vi "Configure RF Output.vi"(4 "Enable Reverse Power Protection (T:Enable)":bool=TRUE, 6 "Enable Blanking (T:Enable)":bool=TRUE, 7 "Enable Modulation (T:Enable)":bool=TRUE, 8 "error in (no error)":errorcluster, 9 "Auto Blanking (T:Enable)":bool=TRUE, 10 "Enable RF Output (F:Disable)":bool, 11 "VISA resource name":refnum<visa-resource-name>) -> (0 "error out":errorcluster, 3 "VISA resource name out":refnum<visa-resource-name>)   [LabVIEW 2012, in "Agilent PSG MXG Series.lvlib"]
doc: "Configures RF output, modulation state, blanking, and RPP circuit of the signal generator."
uses:
  <instrlib>/Agilent PSG MXG Series/Agilent PSG MXG Series.lvlib
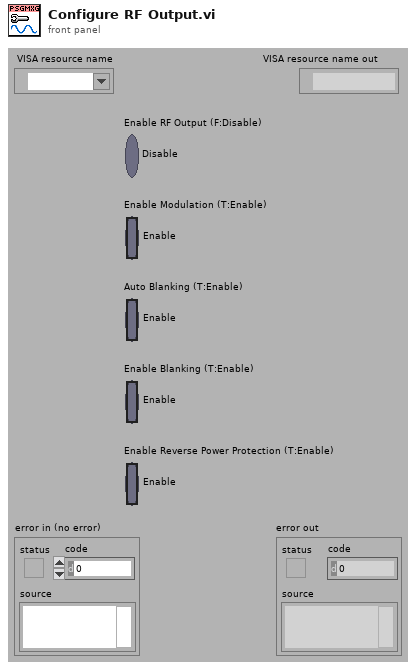
[diagram p1: front panel]
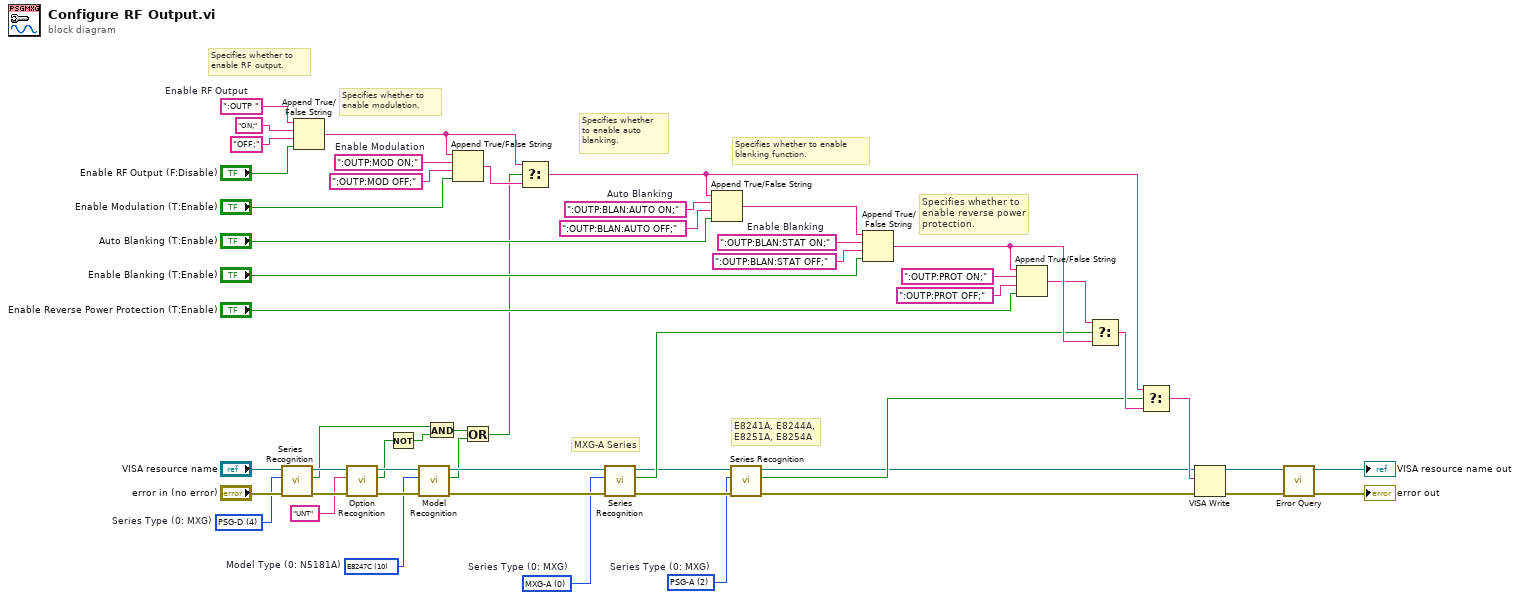
[diagram p0: block diagram]
diagram:
  w1 = u16 4 items=["MXG-A", "PSG", "PSG-A", "PSG-C", "PSG-D", "MXG-B", "EXG"]  # Series Type (0: MXG)
  w2 = u16 10 items=["N5181A"=0, "N5182A"=1, "N5183A"=2, "N5161A"=3, "N5162A"=4, "E8241A"=5, "E8244A"=6, "E8251A"=7, "E8254A"=8, "E8247C"=10, "E8257C"=11, "E8267C"=12, "E8257D"=15, "E8267D"=16, "N5171B"=17, "N5172B"=18, "N5181B"=19, "N5182B"=20]  # Model Type (0: N5181A)
  w3 = u16 2 items=["MXG-A", "PSG", "PSG-A", "PSG-C", "PSG-D", "MXG-B", "EXG"]  # Series Type (0: MXG)
  w4 = u16 0 items=["MXG-A", "PSG", "PSG-A", "PSG-C", "PSG-D", "MXG-B", "EXG"]  # Series Type (0: MXG)
  w31 = ":OUTP:BLAN:STAT ON;"  # Enable Blanking
  w46 = ":OUTP:BLAN:AUTO ON;"  # Auto Blanking
  w49 = ":OUTP:MOD ON;"  # Enable Modulation
  w53 = ":OUTP "  # Enable RF Output
  # "MXG-A Series"
  # "Specifies whether to\nenable reverse power\nprotection."
  # "Specifies whether to enable\nblanking function."
  # "Specifies whether\nto enable auto\nblanking."
  # "Specifies whether to\nenable modulation."
  # "Specifies whether to\nenable RF output."
  # "E8241A, E8244A,\nE8251A, E8254A"
  n1 = call <instrlib>:"Series Recognition.vi"("error in (no error)"="error in (no error)", "Series Type (0: MXG)"=w1, "VISA resource name"="VISA resource name") -> ("error out"=w14:errorcluster, "Is Series Correct"=w8:bool, "VISA resource name out"=w15:refnum<visa-resource-name>)  [unwired: 1 in, 5 out]
  n2 = Append True/False String(1:"Enable RF Output (F:Disable)", 2:"OFF;" ("false string"), 3:"ON;" ("true string"), 4:w53) -> (0:w22:string)
  n3 = call <instrlib>:"Option Recognition.vi"("error in (no error)"=w14, "Option (\"\")"="UNT" ("Option (\"\")"), "VISA resource name"=w15) -> ("error out"=w11:errorcluster, "Is Option Installed"=w10:bool, "VISA resource name out"=w12:refnum<visa-resource-name>)  [unwired: 6 out]
  n4 = Not(x=w10) -> (.not. x?=w9:bool)
  n5 = call <instrlib>:"Model Recognition.vi"("error in (no error)"=w11, "Model Type (0: N5181A)"=w2, "VISA resource name"=w12) -> ("error out"=w18:errorcluster, "Is Model Correct"=w6:bool, "VISA resource name out"=w19:refnum<visa-resource-name>)  [unwired: 6 out]
  n6 = And(x=w8, y=w9) -> (x .and. y?=w7:bool)
  n7 = Append True/False String(1:"Enable Modulation (T:Enable)", 2:":OUTP:MOD OFF;" ("true string"), 3:w49, 4:w22) -> (0:w21:string)
  n8 = Or(x=w7, y=w6) -> (x .or. y?=w5:bool)
  n9 = Select(t=w22, s=w5, f=w21) -> (s? t:f=w20:string)
  n10 = call <instrlib>:"Series Recognition.vi"("error in (no error)"=w18, "Series Type (0: MXG)"=w4, "VISA resource name"=w19) -> ("error out"=w28:errorcluster, "Is Series Correct"=w30:bool, "VISA resource name out"=w29:refnum<visa-resource-name>)  [unwired: 1 in, 5 out]
  n11 = Append True/False String(1:"Auto Blanking (T:Enable)", 2:":OUTP:BLAN:AUTO OFF;" ("true string"), 3:w46, 4:w20) -> (0:w43:string)
  n12 = call <instrlib>:"Series Recognition.vi"("error in (no error)"=w28, "Series Type (0: MXG)"=w3, "VISA resource name"=w29) -> ("error out"=w25:errorcluster, "Is Series Correct"=w27:bool, "VISA resource name out"=w26:refnum<visa-resource-name>)  [unwired: 1 in, 5 out]
  n13 = Append True/False String(1:"Enable Blanking (T:Enable)", 2:":OUTP:BLAN:STAT OFF;" ("true string"), 3:w31, 4:w43) -> (0:w35:string)
  n14 = Append True/False String(1:"Enable Reverse Power Protection (T:Enable)", 2:":OUTP:PROT OFF;" ("true string"), 3:":OUTP:PROT ON;" ("Enable Reverse Power Protection"), 4:w35) -> (0:w34:string)
  n15 = Select(t=w34, s=w30, f=w35) -> (s? t:f=w33:string)
  n16 = Select(t=w20, s=w27, f=w33) -> (s? t:f=w32:string)
  n17 = VISA Write(VISA resource name=w26, write buffer=w32, error in (no error)=w25) -> (VISA resource name out=w37:refnum<visa-resource-name>, error out=w36:errorcluster)  [unwired: 1 out]
  n18 = call <instrlib>:"Error Query.vi"("error in (no error)"=w36, "VISA resource name"=w37) -> ("error out"=→"error out":errorcluster, "VISA resource name out"=→"VISA resource name out":refnum<visa-resource-name>)  [unwired: 8 out]
